vi "gentec-M-Link.Set Wavelength.vi"(0 "VISA resource In":refnum<visa-resource-name>, 2 "Lambda":u16 caption="Wavelength (nm)", 5 "error in (no error)":errorcluster) -> (11 "Data Read":string, 12 "Error":bool, 13 "Read Timeout":bool, 14 "VISA resource Out":refnum<visa-resource-name>, 15 "Min Range":T1 items=["1f", "3f", "10f", "30f", "100f", "300f", "1p", "3p", "10p", "30p", "100p", "300p", "1n", "3n", "10n", "30n", "100n", "300n", "1u", "3u", "10u", "30u", "100u", "300u", "1m", "3m", "10m", "30m", "100m", "300m", "1", "3", "10", "30", "100", "300", "1K", "3K", "10K", "30K", "100K", "300K", "1M", "3M", "10M", "30M", "100M", "300M"], 16 "Max Range":T1 items=["1f", "3f", "10f", "30f", "100f", "300f", "1p", "3p", "10p", "30p", "100p", "300p", "1n", "3n", "10n", "30n", "100n", "300n", "1u", "3u", "10u", "30u", "100u", "300u", "1m", "3m", "10m", "30m", "100m", "300m", "1", "3", "10", "30", "100", "300", "1K", "3K", "10K", "30K", "100K", "300K", "1M", "3M", "10M", "30M", "100M", "300M"], 17 "Current Range":T1 items=["1f", "3f", "10f", "30f", "100f", "300f", "1p", "3p", "10p", "30p", "100p", "300p", "1n", "3n", "10n", "30n", "100n", "300n", "1u", "3u", "10u", "30u", "100u", "300u", "1m", "3m", "10m", "30m", "100m", "300m", "1", "3", "10", "30", "100", "300", "1K", "3K", "10K", "30K", "100K", "300K", "1M", "3M", "10M", "30M", "100M", "300M"], 18 "Corrections":bool, 19 "error out":errorcluster)   [LabVIEW 2014, in "gentec-M-Link - Driver.lvlib"]
doc: "Data to write: wav<n> where <n> is a number\n\nAn error occurs, for example, if the wanted wavelength is out of range."
uses:
  gentec-M-Link - Driver.lvlib
  Type Defs/gentec-M-Link.Range.ctl
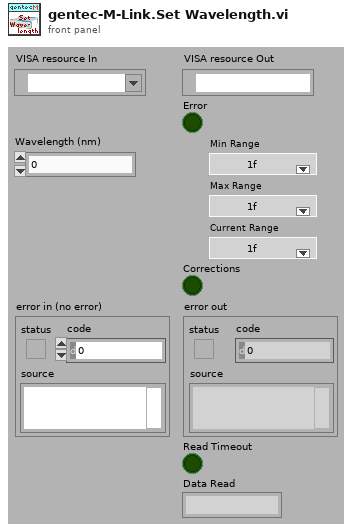
[diagram p1: front panel]
types:
  T1 = typedef "gentec-M-Link - Driver.lvlib/gentec-M-Link.Range.ctl" = u16
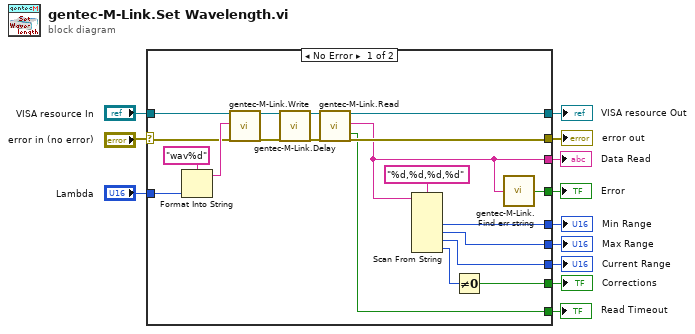
[diagram p0: block diagram]
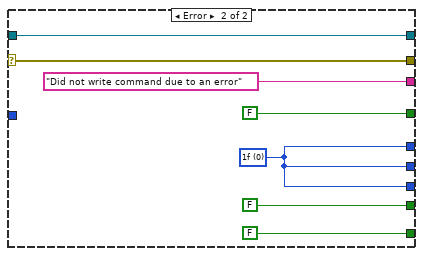
[diagram p2: hidden frame]
diagram:
  n1 = case shown="No Error" "error in (no error)" {
    selector: "error in (no error)" -> [w27 w39]
    tunnel: [w28 w39] -> w11
    tunnel: "VISA resource In" -> [w26 w38]
    tunnel: [w25 w38] -> w9
    tunnel: "Lambda" -> [w24 _]
    tunnel: [w23 FALSE] -> w7
    tunnel: [w22 w37] -> w6
    tunnel: [w21 w37] -> w5
    tunnel: [w20 w37] -> w4
    tunnel: [w19 "Did not write command due to an error" ("Data Read")] -> w3
    tunnel: [w18 FALSE ("Read Timeout")] -> w2
    tunnel: [w17 FALSE ("Found")] -> w1
    frame No Error {
      n2 = Format Into String(format string="wav%d", w24) -> (resulting string=w31:string)  [unwired: 2 in, 1 out]
      n3 = call "gentec-M-Link.Write.vi"("VISA resource (In)"=w26, "Data To Write"=w31, "error in (no error)"=w27) -> ("VISA resource (Out)"=w30:refnum<visa-resource-name>, "error out"=w29:errorcluster)  [unwired: 14 in, 1 out]
      n4 = call "gentec-M-Link.Delay.vi"("VISA resource In"=w30, "error in (no error)"=w29) -> ("VISA resource Out"=w16:refnum<visa-resource-name>, "error out"=w15:errorcluster)  [unwired: 16 in]
      n5 = call "gentec-M-Link.Read.vi"("VISA resource (In)"=w16, "error in (no error)"=w15) -> ("VISA resource (Out)"=w25:refnum<visa-resource-name>, "Data Read"=w19:string, "Read Timeout"=w18:bool, "error out"=w28:errorcluster)  [unwired: 13 in, 1 out]
      n6 = Scan From String(format string="%d,%d,%d,%d", input string=w19) -> (output 1=w20:i32, output 2=w21:i32, output 3=w22:i32, output 4=w13:i32)  [unwired: 6 in, 3 out]
      n7 = Not Equal To 0?(x=w13) -> (x != 0?=w23:bool)
      n8 = call "gentec-M-Link.Find err string.vi"("string"=w19) -> ("Found"=w17:bool)
    }
    frame Error {
      w37 = T1 0 items=["1f", "3f", "10f", "30f", "100f", "300f", "1p", "3p", "10p", "30p", "100p", "300p", "1n", "3n", "10n", "30n", "100n", "300n", "1u", "3u", "10u", "30u", "100u", "300u", "1m", "3m", "10m", "30m", "100m", "300m", "1", "3", "10", "30", "100", "300", "1K", "3K", "10K", "30K", "100K", "300K", "1M", "3M", "10M", "30M", "100M", "300M", "Auto"] ("Min Range")
    }
  }
  "error out" <- w11
  "VISA resource Out" <- w9
  "Corrections" <- w7
  "Current Range" <- w6
  "Max Range" <- w5
  "Min Range" <- w4
  "Data Read" <- w3
  "Read Timeout" <- w2
  "Error" <- w1
